vi "SystemAIFilters.vi"(4 "Lower Cut-Off [Hz]":sgl=1.0 caption="Lower Cut-Off", 6 "Filter Enable":bool, 8 "dt [s]":sgl=0.1 caption="Lower Cut-Off", 11 "SystemAnalogIn":sgl[](array[numeric])) -> (3 "SystemAnalogOut":sgl[](array[numeric]))   [LabVIEW 2016, in "DSI-RT.lvlib"]
uses:
  DSI-RT.lvlib
  <vilib>/Analysis/3filter.llb/Filter Passband Type.ctl
  <vilib>/ptbypt/NI_PtbyPt.lvlib
  <vilib>/Analysis/NI_AALBase.lvlib
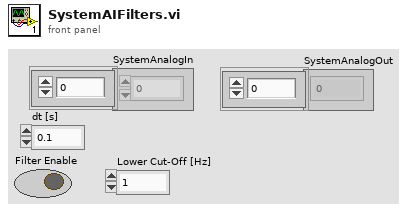
[diagram p1: front panel]
types:
  T1 = typedef "NI_AALBase.lvlib/Filter Passband Type.ctl" = enum32{"Lowpass", "Highpass", "Bandpass", "Bandstop"}
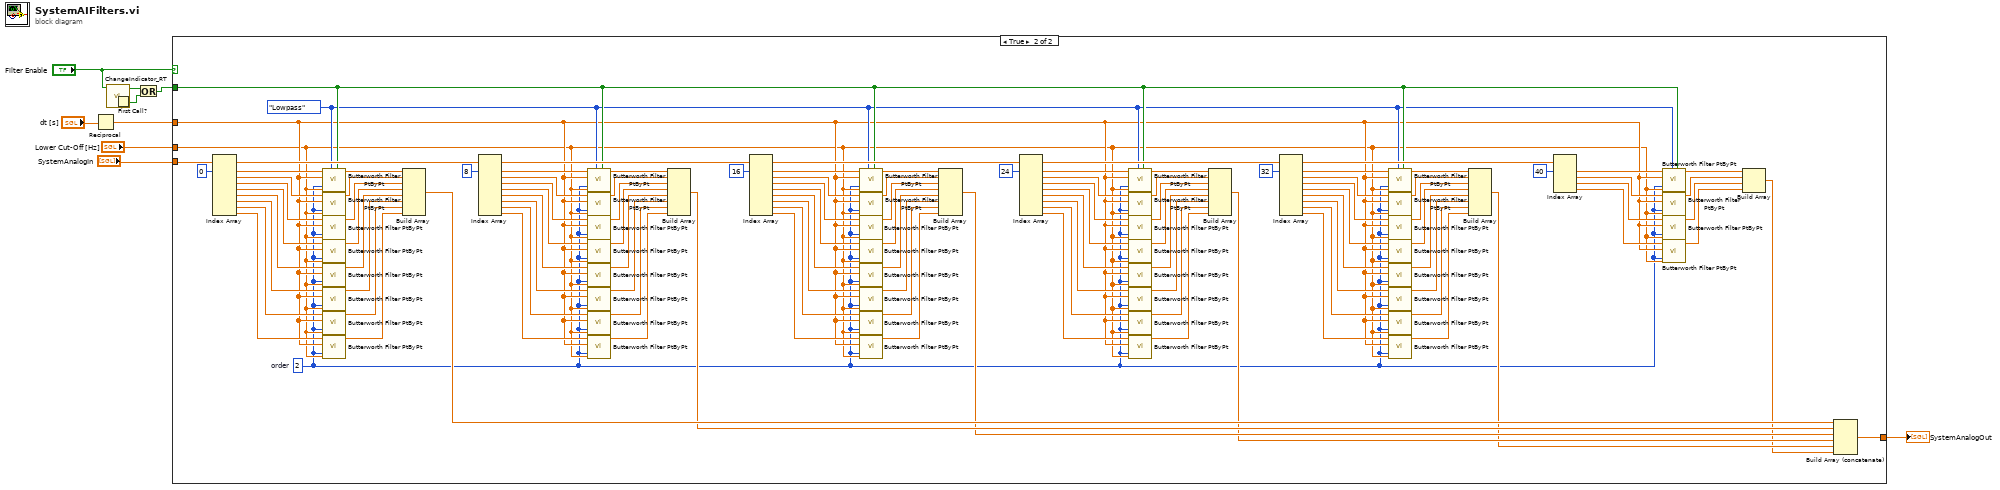
[diagram p0: block diagram]
diagram:
  n1 = Reciprocal(x="dt [s]") -> (1/x=w5:sgl)
  n2 = call "ChangeIndicator_RT.vi"("Input"="Filter Enable") -> ("Change"=w3:bool)  [unwired: 9 in]
  n3 = First Call?() -> (First Call?: T/F=w2:bool)
  n4 = Or(x=w3, y=w2) -> (x .or. y?=w1:bool)
  n5 = case shown="True" "Filter Enable" {
    tunnel: "SystemAnalogIn" -> [w10 w17]
    tunnel: "Lower Cut-Off [Hz]" -> [_ w13]
    tunnel: w1 -> [_ w16]
    tunnel: w5 -> [_ w14]
    tunnel: [w10 w81] -> w4
    frame False {
    }
    frame True {
      w12 = 2  # order
      w15 = Filter_Passband_Type."Lowpass" ("filter type")
      n6 = Index Array(array=w17, index #1=0 ("index")) -> (element #1=w117:sgl, element #2=w116:sgl, element #3=w115:sgl, element #4=w114:sgl, element #5=w113:sgl, element #6=w112:sgl, element #7=w111:sgl, element #8=w110:sgl)  [unwired: 7 in]
      n7 = call <vilib>:"Butterworth Filter PtByPt.vi"("initialize"=w16, "order"=w12, "filter type"=w15, "low cutoff freq: fl"=w13, "sampling freq: fs"=w14, "x"=w117) -> ("Filtered x"=w109:dbl)  [unwired: 3 in, 1 out]
      n8 = call <vilib>:"Butterworth Filter PtByPt.vi"("initialize"=w16, "order"=w12, "filter type"=w15, "low cutoff freq: fl"=w13, "sampling freq: fs"=w14, "x"=w116) -> ("Filtered x"=w108:dbl)  [unwired: 3 in, 1 out]
      n9 = call <vilib>:"Butterworth Filter PtByPt.vi"("initialize"=w16, "order"=w12, "filter type"=w15, "low cutoff freq: fl"=w13, "sampling freq: fs"=w14, "x"=w115) -> ("Filtered x"=w107:dbl)  [unwired: 3 in, 1 out]
      n10 = call <vilib>:"Butterworth Filter PtByPt.vi"("initialize"=w16, "order"=w12, "filter type"=w15, "low cutoff freq: fl"=w13, "sampling freq: fs"=w14, "x"=w114) -> ("Filtered x"=w106:dbl)  [unwired: 3 in, 1 out]
      n11 = call <vilib>:"Butterworth Filter PtByPt.vi"("initialize"=w16, "order"=w12, "filter type"=w15, "low cutoff freq: fl"=w13, "sampling freq: fs"=w14, "x"=w113) -> ("Filtered x"=w105:dbl)  [unwired: 3 in, 1 out]
      n12 = call <vilib>:"Butterworth Filter PtByPt.vi"("initialize"=w16, "order"=w12, "filter type"=w15, "low cutoff freq: fl"=w13, "sampling freq: fs"=w14, "x"=w112) -> ("Filtered x"=w104:dbl)  [unwired: 3 in, 1 out]
      n13 = call <vilib>:"Butterworth Filter PtByPt.vi"("initialize"=w16, "order"=w12, "filter type"=w15, "low cutoff freq: fl"=w13, "sampling freq: fs"=w14, "x"=w111) -> ("Filtered x"=w103:dbl)  [unwired: 3 in, 1 out]
      n14 = call <vilib>:"Butterworth Filter PtByPt.vi"("initialize"=w16, "order"=w12, "filter type"=w15, "low cutoff freq: fl"=w13, "sampling freq: fs"=w14, "x"=w110) -> ("Filtered x"=w102:dbl)  [unwired: 3 in, 1 out]
      n15 = Build Array(w109, w108, w107, w106, w105, w104, w103, w102) -> (w83:dbl[])
      n16 = Index Array(array=w17, index #1=8 ("index")) -> (element #1=w86:sgl, element #2=w87:sgl, element #3=w88:sgl, element #4=w89:sgl, element #5=w90:sgl, element #6=w91:sgl, element #7=w92:sgl, element #8=w93:sgl)  [unwired: 7 in]
      n17 = call <vilib>:"Butterworth Filter PtByPt.vi"("initialize"=w16, "order"=w12, "filter type"=w15, "low cutoff freq: fl"=w13, "sampling freq: fs"=w14, "x"=w86) -> ("Filtered x"=w94:dbl)  [unwired: 3 in, 1 out]
      n18 = call <vilib>:"Butterworth Filter PtByPt.vi"("initialize"=w16, "order"=w12, "filter type"=w15, "low cutoff freq: fl"=w13, "sampling freq: fs"=w14, "x"=w87) -> ("Filtered x"=w95:dbl)  [unwired: 3 in, 1 out]
      n19 = call <vilib>:"Butterworth Filter PtByPt.vi"("initialize"=w16, "order"=w12, "filter type"=w15, "low cutoff freq: fl"=w13, "sampling freq: fs"=w14, "x"=w88) -> ("Filtered x"=w96:dbl)  [unwired: 3 in, 1 out]
      n20 = call <vilib>:"Butterworth Filter PtByPt.vi"("initialize"=w16, "order"=w12, "filter type"=w15, "low cutoff freq: fl"=w13, "sampling freq: fs"=w14, "x"=w89) -> ("Filtered x"=w97:dbl)  [unwired: 3 in, 1 out]
      n21 = call <vilib>:"Butterworth Filter PtByPt.vi"("initialize"=w16, "order"=w12, "filter type"=w15, "low cutoff freq: fl"=w13, "sampling freq: fs"=w14, "x"=w90) -> ("Filtered x"=w98:dbl)  [unwired: 3 in, 1 out]
      n22 = call <vilib>:"Butterworth Filter PtByPt.vi"("initialize"=w16, "order"=w12, "filter type"=w15, "low cutoff freq: fl"=w13, "sampling freq: fs"=w14, "x"=w91) -> ("Filtered x"=w99:dbl)  [unwired: 3 in, 1 out]
      n23 = call <vilib>:"Butterworth Filter PtByPt.vi"("initialize"=w16, "order"=w12, "filter type"=w15, "low cutoff freq: fl"=w13, "sampling freq: fs"=w14, "x"=w92) -> ("Filtered x"=w100:dbl)  [unwired: 3 in, 1 out]
      n24 = call <vilib>:"Butterworth Filter PtByPt.vi"("initialize"=w16, "order"=w12, "filter type"=w15, "low cutoff freq: fl"=w13, "sampling freq: fs"=w14, "x"=w93) -> ("Filtered x"=w101:dbl)  [unwired: 3 in, 1 out]
      n25 = Build Array(w94, w95, w96, w97, w98, w99, w100, w101) -> (w82:dbl[])
      n26 = Index Array(array=w17, index #1=16 ("index")) -> (element #1=w79:sgl, element #2=w78:sgl, element #3=w77:sgl, element #4=w76:sgl, element #5=w75:sgl, element #6=w74:sgl, element #7=w73:sgl, element #8=w72:sgl)  [unwired: 7 in]
      n27 = call <vilib>:"Butterworth Filter PtByPt.vi"("initialize"=w16, "order"=w12, "filter type"=w15, "low cutoff freq: fl"=w13, "sampling freq: fs"=w14, "x"=w79) -> ("Filtered x"=w71:dbl)  [unwired: 3 in, 1 out]
      n28 = call <vilib>:"Butterworth Filter PtByPt.vi"("initialize"=w16, "order"=w12, "filter type"=w15, "low cutoff freq: fl"=w13, "sampling freq: fs"=w14, "x"=w78) -> ("Filtered x"=w70:dbl)  [unwired: 3 in, 1 out]
      n29 = call <vilib>:"Butterworth Filter PtByPt.vi"("initialize"=w16, "order"=w12, "filter type"=w15, "low cutoff freq: fl"=w13, "sampling freq: fs"=w14, "x"=w77) -> ("Filtered x"=w69:dbl)  [unwired: 3 in, 1 out]
      n30 = call <vilib>:"Butterworth Filter PtByPt.vi"("initialize"=w16, "order"=w12, "filter type"=w15, "low cutoff freq: fl"=w13, "sampling freq: fs"=w14, "x"=w76) -> ("Filtered x"=w68:dbl)  [unwired: 3 in, 1 out]
      n31 = call <vilib>:"Butterworth Filter PtByPt.vi"("initialize"=w16, "order"=w12, "filter type"=w15, "low cutoff freq: fl"=w13, "sampling freq: fs"=w14, "x"=w75) -> ("Filtered x"=w67:dbl)  [unwired: 3 in, 1 out]
      n32 = call <vilib>:"Butterworth Filter PtByPt.vi"("initialize"=w16, "order"=w12, "filter type"=w15, "low cutoff freq: fl"=w13, "sampling freq: fs"=w14, "x"=w74) -> ("Filtered x"=w66:dbl)  [unwired: 3 in, 1 out]
      n33 = call <vilib>:"Butterworth Filter PtByPt.vi"("initialize"=w16, "order"=w12, "filter type"=w15, "low cutoff freq: fl"=w13, "sampling freq: fs"=w14, "x"=w73) -> ("Filtered x"=w65:dbl)  [unwired: 3 in, 1 out]
      n34 = call <vilib>:"Butterworth Filter PtByPt.vi"("initialize"=w16, "order"=w12, "filter type"=w15, "low cutoff freq: fl"=w13, "sampling freq: fs"=w14, "x"=w72) -> ("Filtered x"=w64:dbl)  [unwired: 3 in, 1 out]
      n35 = Build Array(w71, w70, w69, w68, w67, w66, w65, w64) -> (w63:dbl[])
      n36 = Index Array(array=w17, index #1=24 ("index")) -> (element #1=w47:sgl, element #2=w48:sgl, element #3=w49:sgl, element #4=w50:sgl, element #5=w51:sgl, element #6=w52:sgl, element #7=w53:sgl, element #8=w54:sgl)  [unwired: 7 in]
      n37 = call <vilib>:"Butterworth Filter PtByPt.vi"("initialize"=w16, "order"=w12, "filter type"=w15, "low cutoff freq: fl"=w13, "sampling freq: fs"=w14, "x"=w47) -> ("Filtered x"=w55:dbl)  [unwired: 3 in, 1 out]
      n38 = call <vilib>:"Butterworth Filter PtByPt.vi"("initialize"=w16, "order"=w12, "filter type"=w15, "low cutoff freq: fl"=w13, "sampling freq: fs"=w14, "x"=w48) -> ("Filtered x"=w56:dbl)  [unwired: 3 in, 1 out]
      n39 = call <vilib>:"Butterworth Filter PtByPt.vi"("initialize"=w16, "order"=w12, "filter type"=w15, "low cutoff freq: fl"=w13, "sampling freq: fs"=w14, "x"=w49) -> ("Filtered x"=w57:dbl)  [unwired: 3 in, 1 out]
      n40 = call <vilib>:"Butterworth Filter PtByPt.vi"("initialize"=w16, "order"=w12, "filter type"=w15, "low cutoff freq: fl"=w13, "sampling freq: fs"=w14, "x"=w50) -> ("Filtered x"=w58:dbl)  [unwired: 3 in, 1 out]
      n41 = call <vilib>:"Butterworth Filter PtByPt.vi"("initialize"=w16, "order"=w12, "filter type"=w15, "low cutoff freq: fl"=w13, "sampling freq: fs"=w14, "x"=w51) -> ("Filtered x"=w59:dbl)  [unwired: 3 in, 1 out]
      n42 = call <vilib>:"Butterworth Filter PtByPt.vi"("initialize"=w16, "order"=w12, "filter type"=w15, "low cutoff freq: fl"=w13, "sampling freq: fs"=w14, "x"=w52) -> ("Filtered x"=w60:dbl)  [unwired: 3 in, 1 out]
      n43 = call <vilib>:"Butterworth Filter PtByPt.vi"("initialize"=w16, "order"=w12, "filter type"=w15, "low cutoff freq: fl"=w13, "sampling freq: fs"=w14, "x"=w53) -> ("Filtered x"=w61:dbl)  [unwired: 3 in, 1 out]
      n44 = call <vilib>:"Butterworth Filter PtByPt.vi"("initialize"=w16, "order"=w12, "filter type"=w15, "low cutoff freq: fl"=w13, "sampling freq: fs"=w14, "x"=w54) -> ("Filtered x"=w62:dbl)  [unwired: 3 in, 1 out]
      n45 = Build Array(w55, w56, w57, w58, w59, w60, w61, w62) -> (w28:dbl[])
      n46 = Index Array(array=w17, index #1=32 ("index")) -> (element #1=w44:sgl, element #2=w43:sgl, element #3=w42:sgl, element #4=w41:sgl, element #5=w40:sgl, element #6=w39:sgl, element #7=w38:sgl, element #8=w37:sgl)  [unwired: 7 in]
      n47 = call <vilib>:"Butterworth Filter PtByPt.vi"("initialize"=w16, "order"=w12, "filter type"=w15, "low cutoff freq: fl"=w13, "sampling freq: fs"=w14, "x"=w44) -> ("Filtered x"=w36:dbl)  [unwired: 3 in, 1 out]
      n48 = call <vilib>:"Butterworth Filter PtByPt.vi"("initialize"=w16, "order"=w12, "filter type"=w15, "low cutoff freq: fl"=w13, "sampling freq: fs"=w14, "x"=w43) -> ("Filtered x"=w35:dbl)  [unwired: 3 in, 1 out]
      n49 = call <vilib>:"Butterworth Filter PtByPt.vi"("initialize"=w16, "order"=w12, "filter type"=w15, "low cutoff freq: fl"=w13, "sampling freq: fs"=w14, "x"=w42) -> ("Filtered x"=w34:dbl)  [unwired: 3 in, 1 out]
      n50 = call <vilib>:"Butterworth Filter PtByPt.vi"("initialize"=w16, "order"=w12, "filter type"=w15, "low cutoff freq: fl"=w13, "sampling freq: fs"=w14, "x"=w41) -> ("Filtered x"=w33:dbl)  [unwired: 3 in, 1 out]
      n51 = call <vilib>:"Butterworth Filter PtByPt.vi"("initialize"=w16, "order"=w12, "filter type"=w15, "low cutoff freq: fl"=w13, "sampling freq: fs"=w14, "x"=w40) -> ("Filtered x"=w32:dbl)  [unwired: 3 in, 1 out]
      n52 = call <vilib>:"Butterworth Filter PtByPt.vi"("initialize"=w16, "order"=w12, "filter type"=w15, "low cutoff freq: fl"=w13, "sampling freq: fs"=w14, "x"=w39) -> ("Filtered x"=w31:dbl)  [unwired: 3 in, 1 out]
      n53 = call <vilib>:"Butterworth Filter PtByPt.vi"("initialize"=w16, "order"=w12, "filter type"=w15, "low cutoff freq: fl"=w13, "sampling freq: fs"=w14, "x"=w38) -> ("Filtered x"=w30:dbl)  [unwired: 3 in, 1 out]
      n54 = call <vilib>:"Butterworth Filter PtByPt.vi"("initialize"=w16, "order"=w12, "filter type"=w15, "low cutoff freq: fl"=w13, "sampling freq: fs"=w14, "x"=w37) -> ("Filtered x"=w29:dbl)  [unwired: 3 in, 1 out]
      n55 = Build Array(w36, w35, w34, w33, w32, w31, w30, w29) -> (w27:dbl[])
      n56 = Index Array(array=w17, index #1=40 ("index")) -> (element #1=w19:sgl, element #2=w20:sgl, element #3=w21:sgl, element #4=w22:sgl)  [unwired: 3 in]
      n57 = call <vilib>:"Butterworth Filter PtByPt.vi"("initialize"=w16, "order"=w12, "filter type"=w15, "low cutoff freq: fl"=w13, "sampling freq: fs"=w14, "x"=w19) -> ("Filtered x"=w23:dbl)  [unwired: 3 in, 1 out]
      n58 = call <vilib>:"Butterworth Filter PtByPt.vi"("initialize"=w16, "order"=w12, "filter type"=w15, "low cutoff freq: fl"=w13, "sampling freq: fs"=w14, "x"=w20) -> ("Filtered x"=w24:dbl)  [unwired: 3 in, 1 out]
      n59 = call <vilib>:"Butterworth Filter PtByPt.vi"("initialize"=w16, "order"=w12, "filter type"=w15, "low cutoff freq: fl"=w13, "sampling freq: fs"=w14, "x"=w21) -> ("Filtered x"=w25:dbl)  [unwired: 3 in, 1 out]
      n60 = call <vilib>:"Butterworth Filter PtByPt.vi"("initialize"=w16, "order"=w12, "filter type"=w15, "low cutoff freq: fl"=w13, "sampling freq: fs"=w14, "x"=w22) -> ("Filtered x"=w26:dbl)  [unwired: 3 in, 1 out]
      n61 = Build Array(w23, w24, w25, w26) -> (w11:dbl[])
      n62 = Build Array (concatenate)(w83, w82, w63, w28, w27, w11) -> (w81:dbl[])
    }
  }
  "SystemAnalogOut" <- w4
